vi "PinoutSettings.vi"() -> ()   [LabVIEW 2023]
panel:
  in  "light-on-threshold":u8=30
  in  "roof-sensor-data-pin":u8=4
  in  "roof-sensor-echo-pin":u8=5
  in  "closed-roof_distance":dbl=3.5
  in  "indoor-light-sensor-pin":u8=3
  in  "outdoor-temp-pin":u8=2
  in  "main-fan-switch-pin":u8=9
  in  "main-light-switch-pin":u8=8
  # "PINOUT"
  # "DIGITAL OUTPUT"
  # "ANALOG INPUT"
  # "SYSTEM SETTINGS"
  # "cm"
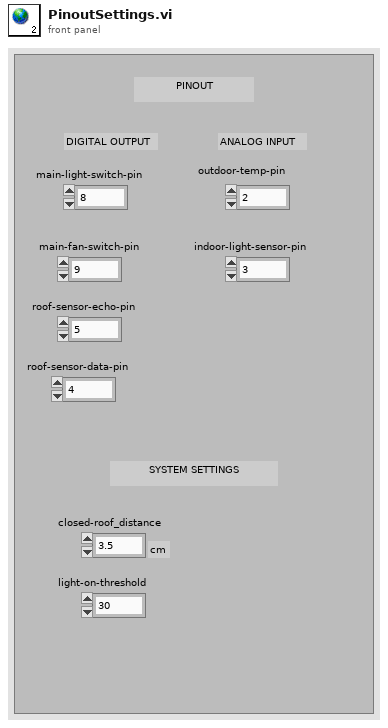
[diagram p1: front panel]
diagram:
